vi "EXEStep Configure UI.vi"(8 "error in (no error)":errorcluster, 10 "Project In":refnum<class "Project.lvclass">, 11 "ConfigureableObject in":refnum<class>) -> (0 "error out":errorcluster, 3 "ConfigureableObject out":refnum<class>)   [LabVIEW 2015, in "CallEXEStep.lvclass"]
uses:
  CallEXEStep.lvclass
  Project.lvclass
  CallEXEStep.lvclass/CallEXEStep.ctl
  Step.lvclass
  Editor/Editor.lvclass
panel:
  in  "Name":string
  in  "Skip":bool
  in  "EXE Path":path
  in  "Arguments":string
  in  "Run Minimized":bool
  in  "Wait Until Completion":bool
  in  "Working Directory":path
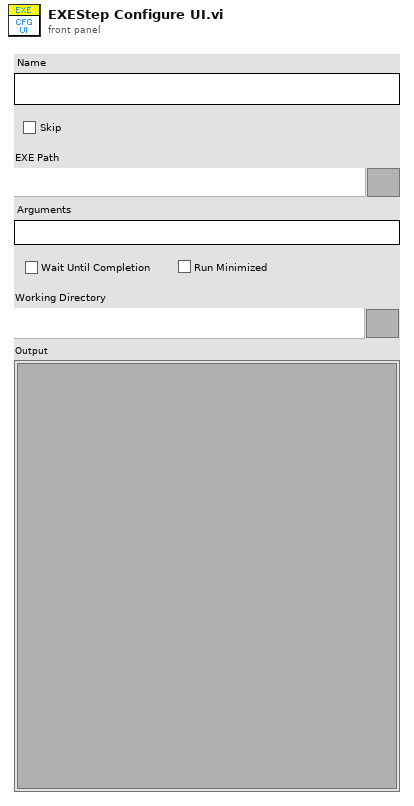
[diagram p1: front panel]
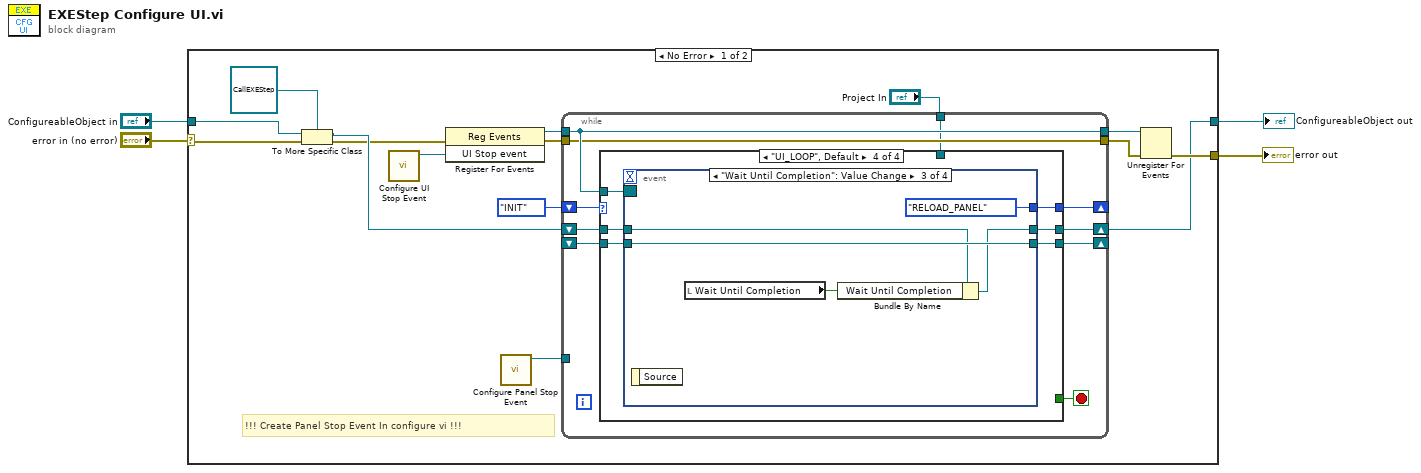
[diagram p0: block diagram]
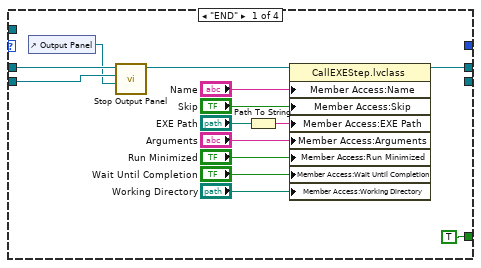
[diagram p2: hidden frame]
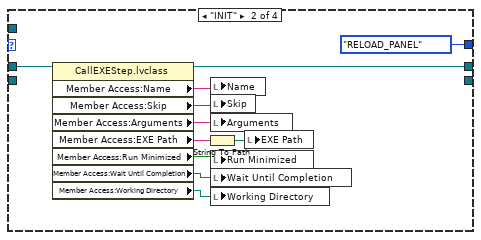
[diagram p3: hidden frame]
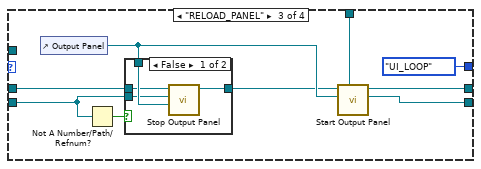
[diagram p4: hidden frame]
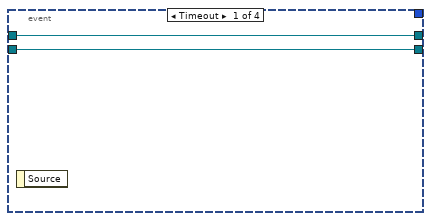
[diagram p6: hidden frame]
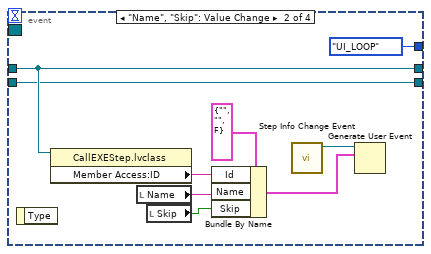
[diagram p7: hidden frame]
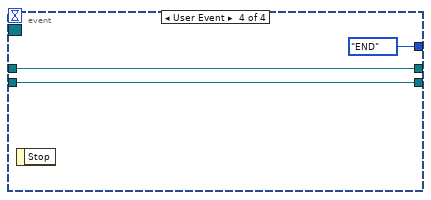
[diagram p8: hidden frame]
diagram:
  n1 = case shown="No Error" "error in (no error)" {
    selector: "error in (no error)" -> [w6 w95]
    tunnel: [w14 w95] -> w3
    tunnel: "ConfigureableObject in" -> [w19 w94]
    tunnel: [w13 w94] -> w1
    frame No Error {
      # "!!! Create Panel Stop Event In configure vi !!!"
      n2 = To More Specific Class(target class=refnum<class "CallEXEStep.lvclass"> refnum ("CallEXEStep.lvclass"), reference=w19, error in=w6) -> (specific class reference=w8:refnum<class "CallEXEStep.lvclass">, error out=w7:errorcluster)
      n3 = call "Configure UI Stop Event.vi"() -> ("UI Stop event"=w9:refnum<user-event>)  [unwired: 11 in]
      n4 = register-events(error in=w7, w9) -> (reference out=w18:refnum<event-registration>, error out=w16:errorcluster)  [unwired: 1 in]
      n5 = call "Configure Panel Stop Event.vi"() -> ("Panel Stop event"=w10:refnum<user-event>)  [unwired: 11 in]
      n6 = while {
        tunnel: w18 -> [w29]
        tunnel: [w29] -> w17
        tunnel: w16 -> [w28]
        tunnel: [w28] -> w15
        shift-right: [w26] -> w13
        shift-left: w8 -> [w27]
        shift-right: [w24] -> _
        shift-left: enum16{"UI_LOOP", "INIT", "END", "RELOAD_PANEL"}."INIT" -> [w25]
        tunnel: w10 -> [_]
        shift-right: [w22] -> _
        shift-left: _ -> [w21]
        tunnel: "Project In" -> [w20]
        stop <- w23 stop-if-true
        n7 = case shown="\"UI_LOOP\", Default" w25 {
          tunnel: w29 -> [_ _ _ w74]
          tunnel: w27 -> [w33 w53 w58 w73]
          tunnel: [w42 w44 w63 w72] -> w26
          tunnel: [_ enum16{"UI_LOOP", "INIT", "END", "RELOAD_PANEL"}."RELOAD_PANEL" enum16{"UI_LOOP", "INIT", "END", "RELOAD_PANEL"}."UI_LOOP" w71] -> w24
          tunnel: [TRUE _ _ _] -> w23
          tunnel: [_ _ w61 w69] -> w22
          tunnel: w21 -> [w31 _ w59 w70]
          tunnel: w20 -> [_ _ w62 _]
          frame "END" {
            n8 = control-ref of="Output Panel"() -> (w30:refnum<vi>)
            n9 = call-dynamic "Stop Output Panel.vi"("Panel Host"=w30, "Panel VI in"=w31, "CallEXEStep in"=w33) -> ("CallEXEStep out"=w32:refnum<class "CallEXEStep.lvclass">)  [unwired: 7 in, 1 out]
            n10 = Path To String(path="EXE Path") -> (string=w40:string)
            n11 = property class="CallEXEStep.lvclass"(reference=w32, "Member Access:Name"="Name", "Member Access:Skip"="Skip", "Member Access:EXE Path"=w40, "Member Access:Arguments"="Arguments", "Member Access:Run Minimized"="Run Minimized", "Member Access:Wait Until Completion"="Wait Until Completion", "Member Access:Working Directory"="Working Directory") -> (reference out=w42:refnum<class "CallEXEStep.lvclass">)  [unwired: 1 in, 1 out]
          }
          frame "INIT" {
            n12 = property class="CallEXEStep.lvclass"(reference=w53) -> (reference out=w44:refnum<class "CallEXEStep.lvclass">, "Member Access:Name"=w52:string, "Member Access:Skip"=w51:bool, "Member Access:Arguments"=w45:string, "Member Access:EXE Path"=w50:string, "Member Access:Run Minimized"=w48:bool, "Member Access:Wait Until Completion"=w47:bool, "Member Access:Working Directory"=w46:path)  [unwired: 1 in, 1 out]
            n13 = String To Path(string=w50) -> (path=w49:path)
            n14 = local write "Name"(w52) -> ()
            n15 = local write "Skip"(w51) -> ()
            n16 = local write "Arguments"(w45) -> ()
            n17 = local write "Run Minimized"(w48) -> ()
            n18 = local write "Wait Until Completion"(w47) -> ()
            n19 = local write "Working Directory"(w46) -> ()
            n20 = local write "EXE Path"(w49) -> ()
          }
          frame "RELOAD_PANEL" {
            n21 = control-ref of="Output Panel"() -> (w60:refnum<vi>)
            n22 = Not A Number/Path/Refnum?(number/path/refnum=w59) -> (NaN/Path/Refnum?=w56:bool)
            n23 = case shown="False" w56 {
              tunnel: w60 -> [w67 _]
              tunnel: w59 -> [w66 _]
              tunnel: w58 -> [w65 w68]
              tunnel: [w64 w68] -> w57
              frame False {
                n24 = call-dynamic "Stop Output Panel.vi"("Panel Host"=w67, "Panel VI in"=w66, "CallEXEStep in"=w65) -> ("CallEXEStep out"=w64:refnum<class "CallEXEStep.lvclass">)  [unwired: 7 in, 1 out]
              }
              frame True {
              }
            }
            n25 = call-dynamic "Start Output Panel.vi"("Project In"=w62, "Panel Hostl Refnum"=w60, "CallEXEStep in"=w57) -> ("Panel VI Refnum"=w61:refnum<vi>, "CallEXEStep out"=w63:refnum<class "CallEXEStep.lvclass">)  [unwired: 6 in, 1 out]
          }
          frame "UI_LOOP", Default {
            n26 = event shown="[2] \"Wait Until Completion\": Value Change" {
              selector: w74 -> [_ _ _ _]
              dyn-events: _ -> [_ _ _ _]
              timeout: _ -> [_ _ _ _]
              tunnel: w73 -> [w76 w80 w88 w93]
              tunnel: [w76 w80 w87 w93] -> w72
              tunnel: [_ enum16{"UI_LOOP", "INIT", "END", "RELOAD_PANEL"}."UI_LOOP" enum16{"UI_LOOP", "INIT", "END", "RELOAD_PANEL"}."RELOAD_PANEL" enum16{"UI_LOOP", "INIT", "END", "RELOAD_PANEL"}."END"] -> w71
              tunnel: w70 -> [w75 w79 w90 w91]
              tunnel: [w75 w79 w90 w91] -> w69
              event Timeout {
                n27 = event-data() -> ()  [unwired: 1 in, 1 out]
              }
              event "Name", "Skip": Value Change {
                n28 = event-data() -> ()  [unwired: 1 in, 1 out]
                n29 = property class="CallEXEStep.lvclass"(reference=w80) -> ("Member Access:ID"=w83:string)  [unwired: 1 in, 2 out]
                n30 = local read "Name"() -> (w78:string)
                n31 = local read "Skip"() -> (w77:bool)
                n32 = Bundle By Name(cluster=cluster{"Id":string, "Name":string, "Skip":bool} {"Id"="", "Name"="", "Skip"=FALSE} ("Step Info"), "Id"=w83, "Name"=w78, "Skip"=w77) -> (w85:cluster{"Id":string, "Name":string, "Skip":bool})
                n33 = call "Step Info Change Event.vi"() -> ("Step Info Change Event"=w82:refnum<user-event>)  [unwired: 11 in]
                n34 = Generate User Event(user event=w82, event data cluster=w85) -> ()  [unwired: 2 in, 2 out]
              }
              event "Wait Until Completion": Value Change {
                n35 = event-data() -> ()  [unwired: 1 in, 1 out]
                n36 = local read "Wait Until Completion"() -> (w86:bool)
                n37 = Bundle By Name(cluster=w88, "Wait Until Completion"=w86) -> (w87:refnum<class "CallEXEStep.lvclass">)
              }
              event User Event {
                n38 = event-data() -> ()  [unwired: 1 in, 1 out]
              }
            }
          }
        }
      }
      n39 = Unregister For Events(event registration refnum=w17, error in=w15) -> (error out=w14:errorcluster)
    }
    frame Error {
    }
  }
  "error out" <- w3
  "ConfigureableObject out" <- w1
